vi "Write pipette counter.vi"(8 "error in (no error)":errorcluster, 10 "pipette counter":dbl, 11 "Pipette in":refnum<class "Pipette.lvclass">) -> (0 "error out":errorcluster, 3 "Pipette out":refnum<class "Pipette.lvclass">)   [LabVIEW 2018, in "Pipette.lvclass"]
uses:
  Pipette.lvclass
  Pipette.lvclass/Pipette.ctl
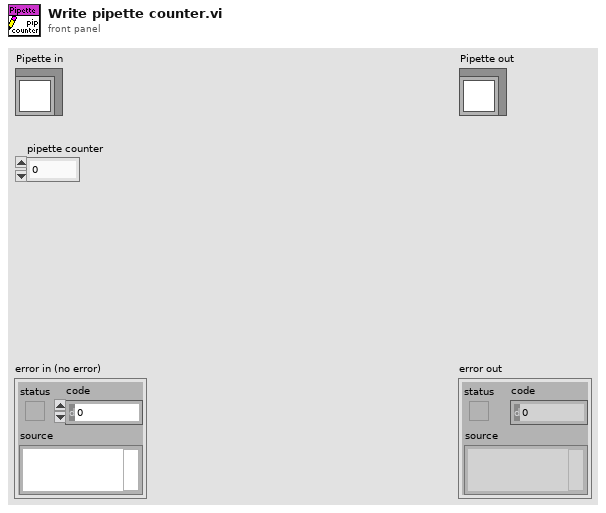
[diagram p1: front panel]
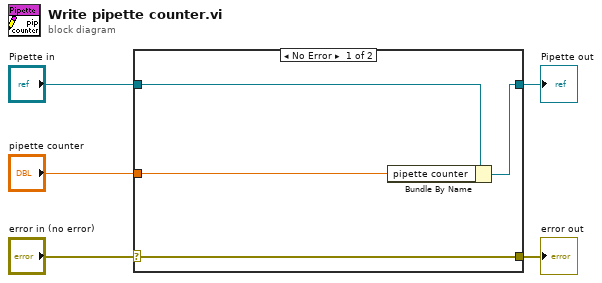
[diagram p0: block diagram]
diagram:
  n1 = case shown="No Error" "error in (no error)" {
    selector: "error in (no error)" -> [w9 w10]
    tunnel: [w9 w10] -> w4
    tunnel: [w7 w11] -> w2
    tunnel: "Pipette in" -> [w8 w11]
    tunnel: "pipette counter" -> [w6 _]
    frame No Error {
      n2 = Bundle By Name(cluster=w8, "pipette counter"=w6) -> (w7:refnum<class "Pipette.lvclass">)
    }
    frame Error {
    }
  }
  "error out" <- w4
  "Pipette out" <- w2
